vi "writeI32.vi"(8 "error in (no error)":errorcluster, 9 "Timeout":i32, 10 "Data":i32[](array[numeric]), 11 "IWriteFIFO in":refnum<class "IWriteFIFO.lvclass">) -> (0 "error out":errorcluster, 2 "ElementsRemaining":u32, 3 "IWriteFIFO out":refnum<class "IWriteFIFO.lvclass">)   [LabVIEW 2015, in "RTFPGA.lvlib" / "IWriteFIFO.lvclass"]
uses:
  IWriteFIFO.lvclass
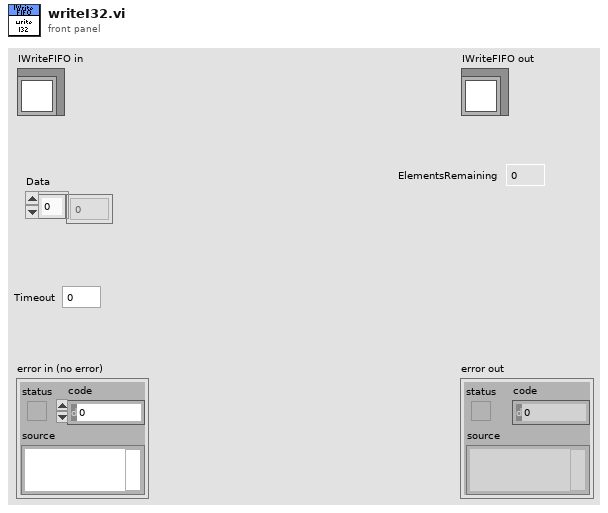
[diagram p1: front panel]
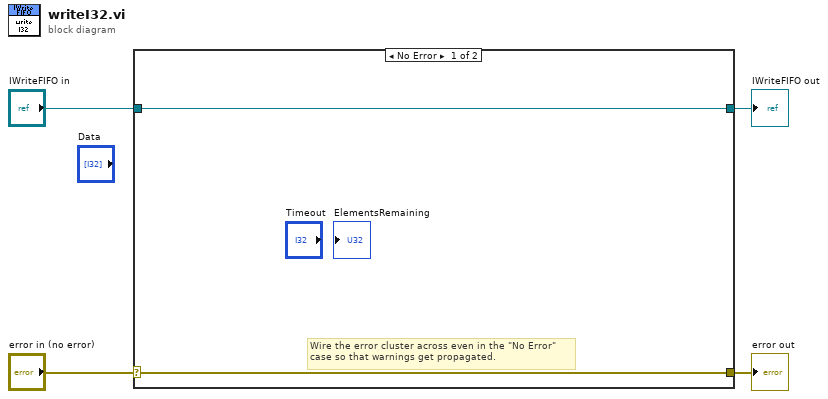
[diagram p0: block diagram]
diagram:
  n1 = case shown="No Error" "error in (no error)" {
    selector: "error in (no error)" -> [w5 w8]
    tunnel: [w5 w8] -> w3
    tunnel: [w6 w7] -> w1
    tunnel: "IWriteFIFO in" -> [w6 w7]
    frame No Error {
      # "Wire the error cluster across even in the \"No Error\"\ncase so that warnings get propagated."
    }
    frame Error {
    }
  }
  "error out" <- w3
  "IWriteFIFO out" <- w1
